vi "PQftablecol.vi"(8 "error in (no error)":errorcluster, 10 "field_num":u32, 11 "res":u32) -> (0 "error out":errorcluster, 2 "table_column_number":i32, 3 "res_out":u32)   [LabVIEW 2019, in "libpqlv.lvlib"]
doc: "Returns the column number (within its table) of the column making up the specified query result column. Query-result column numbers start at 0, but table columns have nonzero numbers.\nZero is returned if the column number is out of range, or if the specified column is not a simple reference to a table column, or when using pre-3.0 protocol."
uses:
  libpqlv.lvlib
  libpq.dll
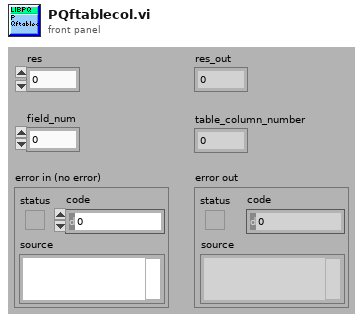
[diagram p1: front panel]
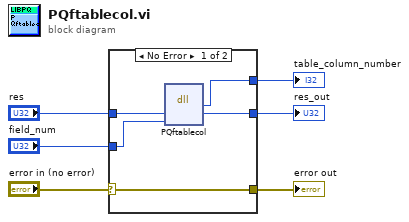
[diagram p0: block diagram]
diagram:
  n1 = case shown="No Error" "error in (no error)" {
    selector: "error in (no error)" -> [w11 w13]
    tunnel: [w11 w13] -> w5
    tunnel: [w10 _] -> w4
    tunnel: "field_num" -> [w9 _]
    tunnel: "res" -> [w8 w12]
    tunnel: [w7 w12] -> w1
    frame No Error {
      n2 = dll-call lib="libpq.*" fn="PQftablecol"("res"=w8, "field_num"=w9) -> ("table_column_number"=w10:i32, "res"=w7:u32)  [unwired: 4 in, 2 out]
    }
    frame Error {
    }
  }
  "table_column_number" <- w4
  "error out" <- w5
  "res_out" <- w1
